vi "Send Drag Event.vi"(8 "error in (no error)":errorcluster, 9 "Horizontal":i32, 10 "Vertical":i32, 11 "QMenu Class in":refnum<class "QMenu Class.lvclass">) -> (0 "error out":errorcluster, 2 "Confirm":bool, 3 "QMenu Class out":refnum<class "QMenu Class.lvclass">)   [LabVIEW 2020, in "QTab.lvlib" / "QMenu Class.lvclass"]
uses:
  QMenu Class.lvclass
  QMenu Class.lvclass/QMenu Class.ctl
  Drag Event Data.ctl
  Read Drag Timeout.vi
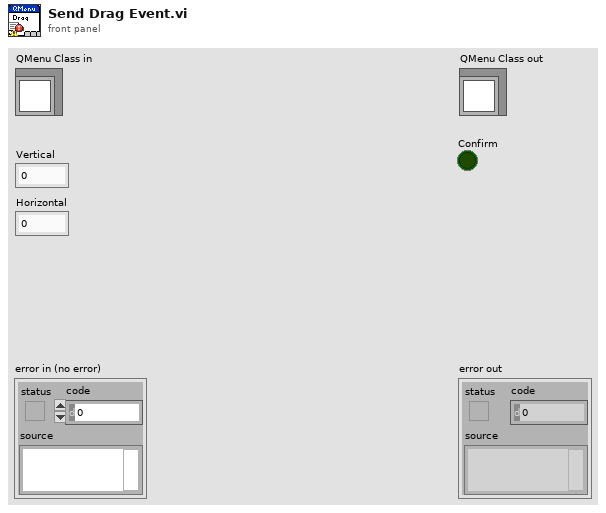
[diagram p1: front panel]
types:
  T1 = typedef "QTab.lvlib/QMenu Class.lvclass/Button Attribute.ctl" = cluster{"Label":string, "Button Text":string, "Closable":bool, "Draggable":bool}
  T2 = typedef "QTab.lvlib/QMenu Class.lvclass/Drag Event Data.ctl" = cluster{"Index":i32, "Label":string, "Vertical":i32, "Horizontal":i32, "Confirm Notifier":refnum<notifier>}
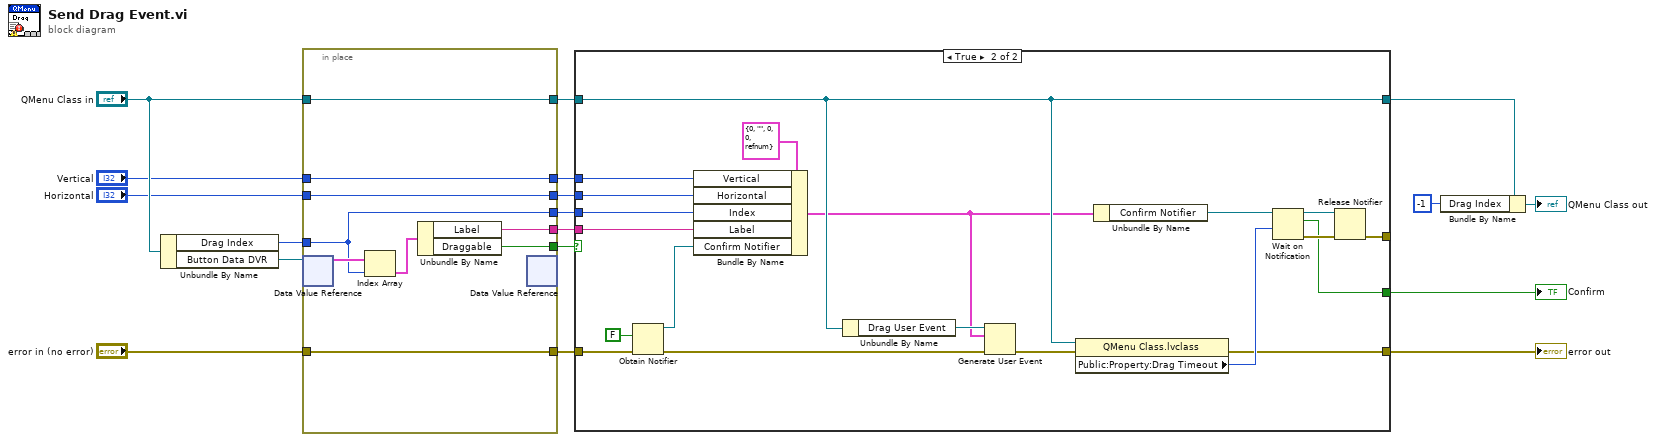
[diagram p0: block diagram]
diagram:
  n1 = Unbundle By Name("QMenu Class in") -> ("Drag Index"=w15:i32, "Button Data DVR"=w18:refnum<data-value>)
  n2 = in-place {
    in-place-border: w15 -> [w21]
    in-place-border: "error in (no error)" -> [w25]
    in-place-border: "QMenu Class in" -> [w24]
    in-place-border: [w24] -> w13
    in-place-border: [w25] -> w14
    in-place-border: [w23] -> w12
    in-place-border: [w22] -> w11
    in-place-border: [w21] -> w10
    in-place-border: "Vertical" -> [w20]
    in-place-border: [w20] -> w4
    in-place-border: "Horizontal" -> [w19]
    in-place-border: [w19] -> w2
    n3 = in-place-dvr #1(w18) -> (w27:T1[])  [unwired: 1 out]
    n4 = Index Array(array=w27, index=w21) -> (element=w26:T1)
    n5 = Unbundle By Name(w26) -> ("Label"=w22:string, "Draggable"=w23:bool)
    n6 = in-place-dvr #1() -> ()  [unwired: 1 in, 2 out]
  }
  n7 = case shown="True" w12 {
    tunnel: w13 -> [w28 w38]
    tunnel: w14 -> [w29 w42]
    tunnel: w10 -> [_ w48]
    tunnel: w11 -> [_ w47]
    tunnel: [w29 w31] -> w6
    tunnel: [w28 w38] -> w9
    tunnel: w4 -> [_ w45]
    tunnel: w2 -> [_ w44]
    tunnel: [_ w32] -> _
    tunnel: [_ w30] -> w1
    frame False {
    }
    frame True {
      n8 = Obtain Notifier(notification data type=FALSE, error in (no error)=w42) -> (notifier out=w41:refnum<notifier>, error out=w40:errorcluster)  [unwired: 2 in, 1 out]
      n9 = Bundle By Name(cluster=T2 {"Index"=0, "Label"="", "Vertical"=0, "Horizontal"=0, "Confirm Notifier"=refnum} ("Drag Event Data"), "Vertical"=w45, "Horizontal"=w44, "Index"=w48, "Label"=w47, "Confirm Notifier"=w41) -> (w37:T2)
      n10 = Unbundle By Name(w38) -> ("Drag User Event"=w49:refnum<user-event>)
      n11 = Generate User Event(user event=w49, event data cluster=w37, error in=w40) -> (error out=w39:errorcluster)  [unwired: 1 in, 1 out]
      n12 = property class="QMenu Class.lvclass"(reference=w38, error in=w39) -> (error out=w31:errorcluster, "Public:Property:Drag Timeout"=w33:i32)  [unwired: 1 out]
      n13 = Unbundle By Name(w37) -> ("Confirm Notifier"=w36:refnum<notifier>)
      n14 = Wait on Notification(notifier=w36, timeout in ms (-1)=w33) -> (notifier out=w35:refnum<notifier>, notification=w30:bool, error out=w34:errorcluster)  [unwired: 2 in, 1 out]
      n15 = Release Notifier(notifier=w35, error in (no error)=w34) -> (error out=w32:errorcluster)  [unwired: 1 in, 2 out]
    }
  }
  "error out" <- w6
  "Confirm" <- w1
  n16 = Bundle By Name(cluster=w9, "Drag Index"=-1 ("Buffer Data.Drag Index")) -> (→"QMenu Class out":refnum<class "QMenu Class.lvclass">)
